vi "Generate_WayPoints_Hopping_LineScan.vi"(11 "Input Cluster":T2={"Scan Rate (um/s)"=15.0, "X Start"=15.0, "X End"=15.0, "Y Start"=15.0, "Y End"=15.0, " Z Start"=15.0, "HoppingDistance"=1.0, "V"=15.0, "Z End"=15.0, "Approach Rate Hopping (um/s)"=15.0, "Retract Rate (um/s)"=15.0, "V 2"=15.0, "Approach Rate (um/s)"=15.0}) -> (0 "output cluster":T1)   [LabVIEW 2023]
uses:
  TypeDefs/WayPointCluster.ctl
  User_Vi/Settings.vi
panel:
  out "Numeric":i32
  in  "WayPointCluster":T1
  out "Y  P":dbl
  out "X  P":dbl
  out "HoppingDistanceX":dbl
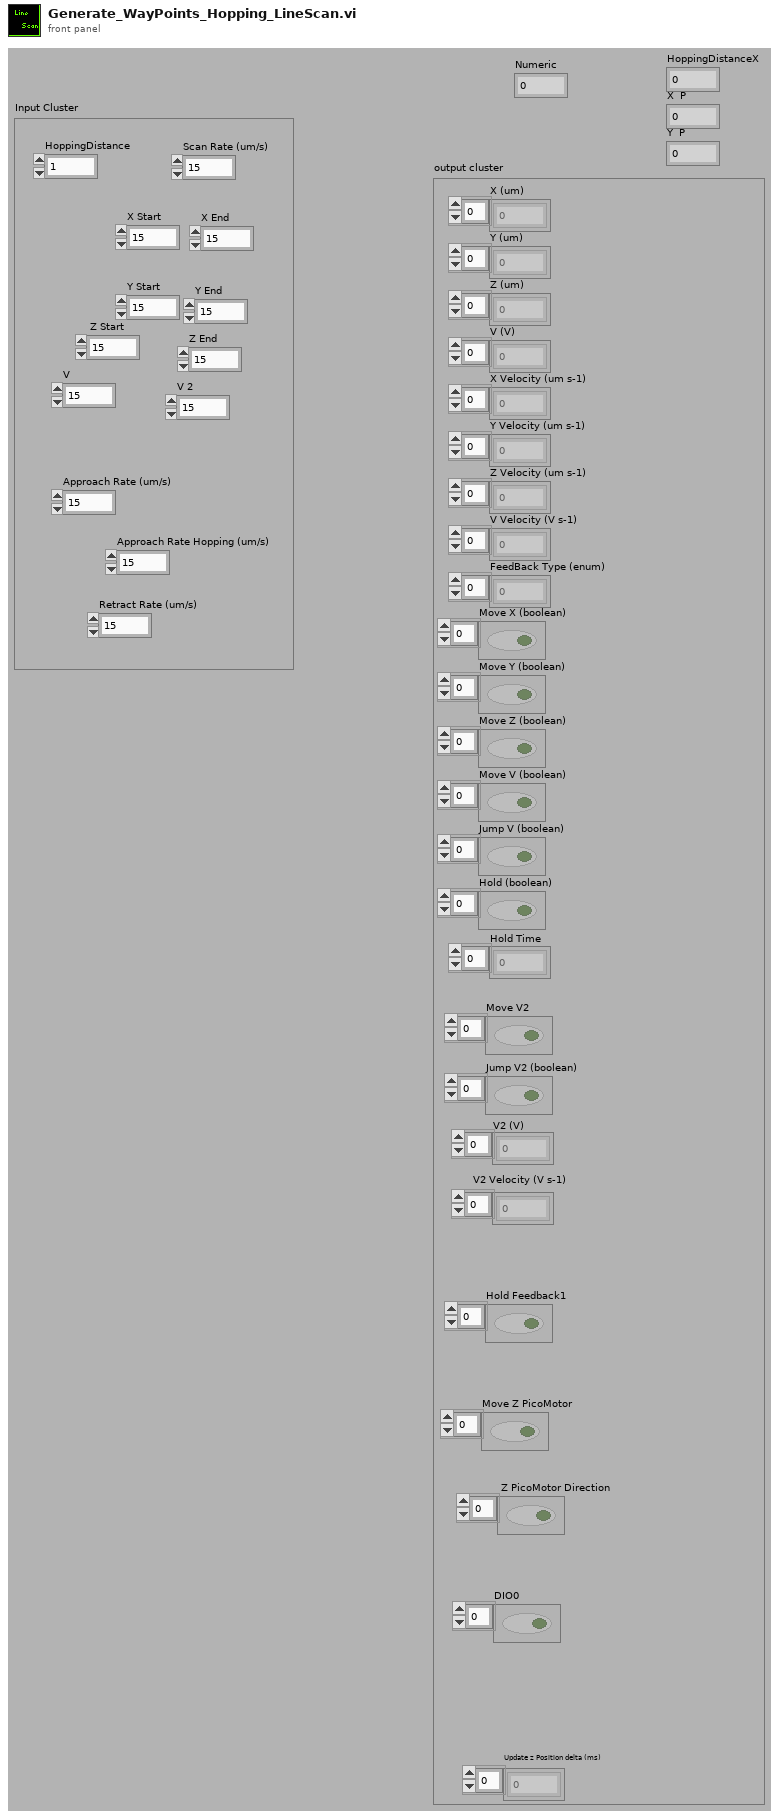
[diagram p1: front panel]
types:
  T1 = typedef "WayPointCluster.ctl" = cluster{"X (um)":dbl[], "Y (um)":dbl[], "Z (um)":dbl[], "V (V)":dbl[], "X Velocity (um s-1)":dbl[], "Y Velocity (um s-1)":dbl[], "Z Velocity (um s-1)":dbl[], "V Velocity (V s-1)":dbl[], "FeedBack Type (enum)":u16[], "Move X (boolean)":bool[], "Move Y (boolean)":bool[], "Move Z (boolean)":bool[], "Move V (boolean)":bool[], "Jump V (boolean)":bool[], "Hold (boolean)":bool[], "Hold Time":u32[], "V2 (V)":dbl[], "Move V2":bool[], "V2 Velocity (V s-1)":dbl[], "Jump V2 (boolean)":bool[], "Update z Position delta (ms)":i16[], "Hold Feedback1":bool[], "Move Z PicoMotor":bool[], " Z PicoMotor Direction":bool[], "DIO0":bool[]}
  T2 = cluster{"Scan Rate (um/s)":dbl, "X Start":dbl, "X End":dbl, "Y Start":dbl, "Y End":dbl, " Z Start":dbl, "HoppingDistance":dbl, "V":dbl, "Z End":dbl, "Approach Rate Hopping (um/s)":dbl, "Retract Rate (um/s)":dbl, "V 2":dbl, "Approach Rate (um/s)":dbl}
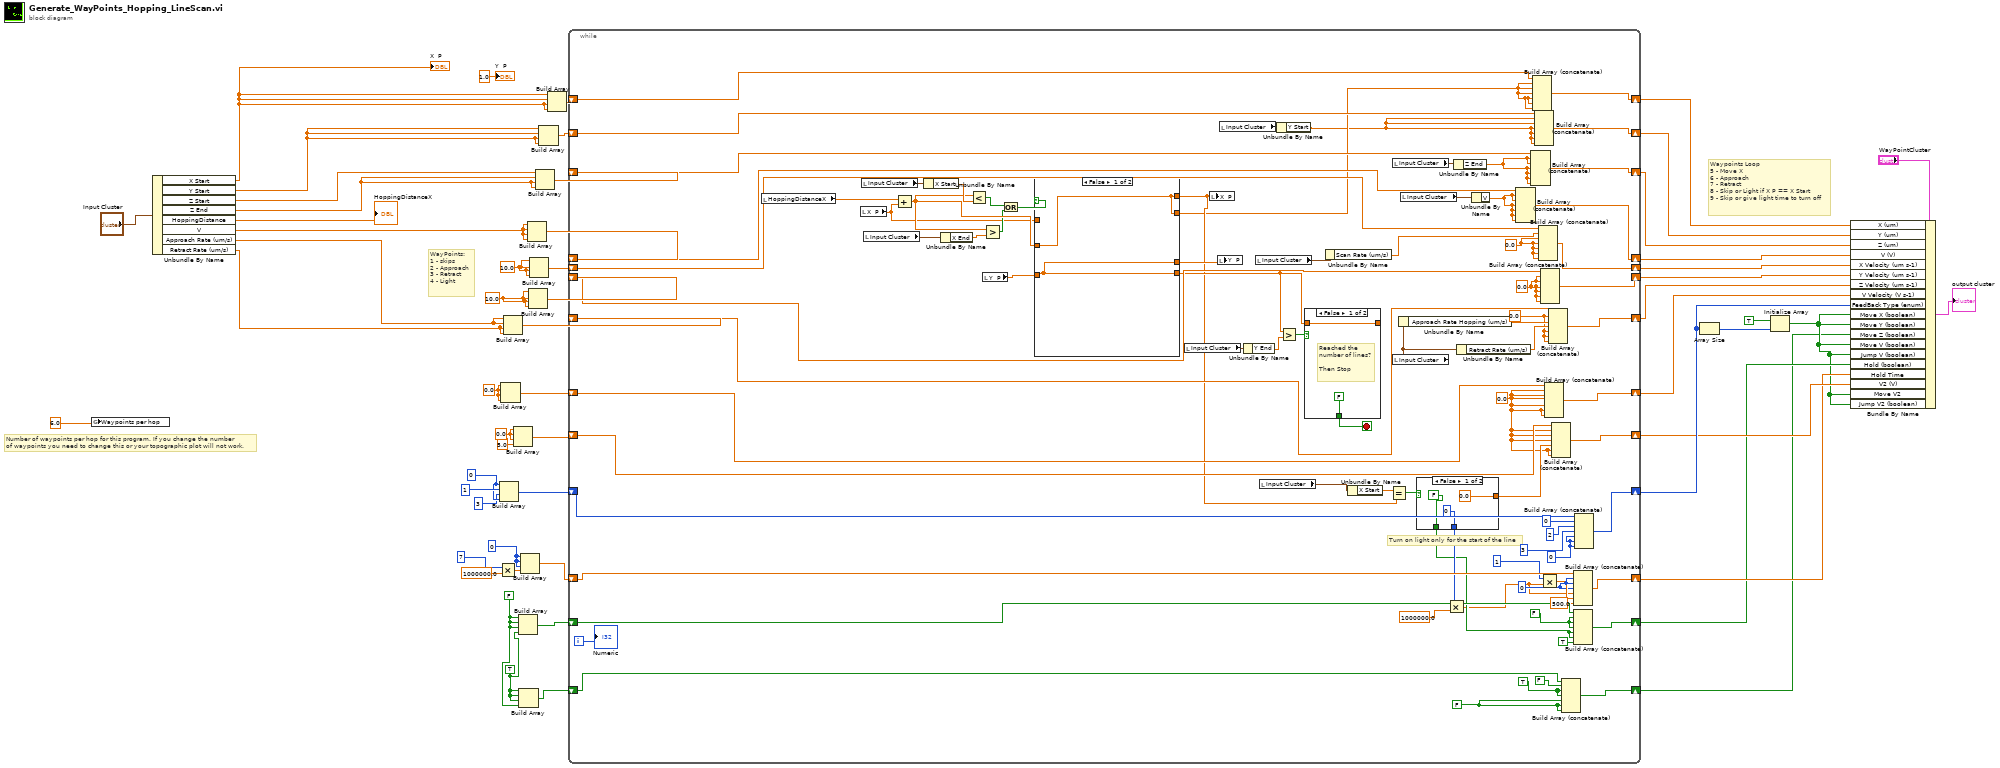
[diagram p0: block diagram]
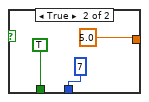
[diagram p2: hidden frame]
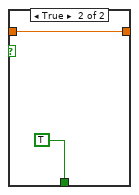
[diagram p3: hidden frame]
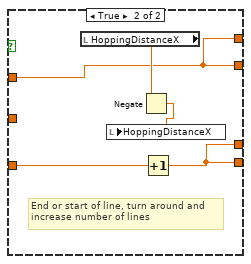
[diagram p4: hidden frame]
diagram:
  w19 = TRUE
  w20 = FALSE
  w28 = u16 0 ("element")
  w16 = 0.0 ("element")
  w17 = u16 0 ("element")
  w12 = 10.0 ("element")
  w13 = 10.0 ("element")
  w15 = 0.0 ("element")
  # "Number of waypoints per hop for this program. If you change the number\nof waypoints you need to change this or your topographic plot will not work."
  # "Waypoints Loop\n5 - Move X\n6 - Approach\n7 - Retract\n8 - Skip or Light if X P == X Start\n9 - Skip or give light time to turn off"
  # "WayPoints:\n1 - skips\n2 - Approach\n3 - Retract\n4 - Light"
  n1 = global write "Settings.vi" "Waypoints per hop"(6.0) -> ()
  n2 = Unbundle By Name("Input Cluster") -> ("X Start"=w8:dbl, "Y Start"=w7:dbl, "Z Start"=w37:dbl, "Z End"=w9:dbl, "HoppingDistance"=→"HoppingDistanceX":dbl, "V"=w11:dbl, "Approach Rate (um/s)"=w34:dbl, "Retract Rate (um/s)"=w14:dbl)
  "X  P" <- w8
  n3 = Multiply(x=u16 7 ("element"), y=1000000.0) -> (x*y=w18:dbl)
  n4 = Build Array(w17, u16 1 ("element"), u16 3 ("element"), w17) -> (w40:u16[])
  n5 = Build Array(w15, w15, w15, w15) -> (w30:dbl[])
  n6 = Build Array(w34, w34, w14, w14) -> (w43:dbl[])
  n7 = Build Array(w16, w16, w16, 5.0 ("element")) -> (w29:dbl[])
  n8 = Build Array(w20, w20, w20, w19) -> (w24:bool[])
  n9 = Build Array(w19, w19, w19, w20) -> (w22:bool[])
  n10 = Build Array(w28, w28, w28, w18) -> (w27:dbl[])
  n11 = Build Array(w11, w11, w11, w11) -> (w48:dbl[])
  n12 = Build Array(w13, w13, w13, w13) -> (w45:dbl[])
  n13 = Build Array(w12, w12, w12, w12) -> (w46:dbl[])
  n14 = Build Array(w37, w9, w9, w9) -> (w50:dbl[])
  n15 = Build Array(w7, w7, w7, w7) -> (w51:dbl[])
  n16 = Build Array(w8, w8, w8, w8) -> (w53:dbl[])
  n17 = while {
    shift-right: [w135] -> w52
    shift-left: w53 -> [w136]
    shift-right: [w127] -> w38
    shift-left: w51 -> [w118]
    shift-right: [w126] -> w49
    shift-left: w50 -> [w134]
    shift-right: [w125] -> w47
    shift-left: w48 -> [w133]
    shift-right: [w124] -> w4
    shift-left: w46 -> [w132]
    shift-right: [w100] -> w44
    shift-left: w45 -> [w131]
    shift-right: [w123] -> w42
    shift-left: w43 -> [w130]
    shift-right: [w122] -> w41
    shift-left: w30 -> [w129]
    shift-right: [w121] -> w36
    shift-left: w40 -> [w128]
    shift-right: [w95] -> w31
    shift-left: w29 -> [w90]
    shift-right: [w88] -> w26
    shift-left: w27 -> [w89]
    shift-right: [w87] -> w25
    shift-left: w24 -> [w85]
    shift-right: [w81] -> w21
    shift-left: w22 -> [w80]
    i -> [w83]
    stop <- w108 stop-if-true
    w60 = u16 0 ("element")
    w57 = FALSE
    w82 = TRUE
    w86 = FALSE
    w75 = u16 0 ("element")
    w63 = 0.0 ("element")
    w64 = 0.0 ("element")
    w61 = 0.0 ("element")
    w62 = 0.0 ("element")
    # "Turn on light only for the start of the line"
    n18 = local read "HoppingDistanceX"() -> (w101:dbl)
    n19 = local read "X  P"() -> (w102:dbl)
    n20 = local read "Input Cluster"() -> (w138:T2)
    n21 = local read "Input Cluster"() -> (w137:T2)
    n22 = Add(x=w101, y=w102) -> (x+y=w114:dbl)
    n23 = Unbundle By Name(w138) -> ("X Start"=w117:dbl)
    n24 = Unbundle By Name(w137) -> ("X End"=w115:dbl)
    n25 = Less?(x=w114, y=w117) -> (x < y?=w116:bool)
    n26 = local read "Y  P"() -> (w74:dbl)
    n27 = Greater?(x=w114, y=w115) -> (0:w113:bool)
    n28 = Or(x=w116, y=w113) -> (x .or. y?=w112:bool)
    n29 = case shown="False" w112 {
      tunnel: w114 -> [w150 _]
      tunnel: [w150 w153] -> w68
      tunnel: w102 -> [_ w153]
      tunnel: [w149 w152] -> w107
      tunnel: [w149 w152] -> w106
      tunnel: [w150 w153] -> w79
      tunnel: w74 -> [w149 w151]
      frame False {
      }
      frame True {
        # "End or start of line, turn around and \nincrease number of lines"
        n30 = local read "HoppingDistanceX"() -> (w155:dbl)
        n31 = Negate(x=w155) -> (-x=w154:dbl)
        n32 = local write "HoppingDistanceX"(w154) -> ()
        n33 = Increment(x=w151) -> (x+1=w152:dbl)
      }
    }
    n34 = local read "Input Cluster"() -> (w111:T2)
    n35 = local write "X  P"(w79) -> ()
    n36 = local write "Y  P"(w106) -> ()
    n37 = local read "Input Cluster"() -> (w96:T2)
    n38 = Unbundle By Name(w111) -> ("Y End"=w110:dbl)
    n39 = local read "Input Cluster"() -> (w70:T2)
    n40 = local read "Input Cluster"() -> (w93:T2)
    n41 = Unbundle By Name(w96) -> ("Y Start"=w67:dbl)
    n42 = Greater?(x=w107, y=w110) -> (0:w109:bool)
    n43 = case shown="False" w109 {
      tunnel: w107 -> [w146 w148]
      tunnel: [w146 w148] -> _
      tunnel: [FALSE TRUE] -> w108
      frame False {
        # "Reached the \nnumber of lines?\n\nThen Stop"
      }
      frame True {
      }
    }
    n44 = Unbundle By Name(w70) -> ("Scan Rate (um/s)"=w69:dbl)
    n45 = Unbundle By Name(w93) -> ("X Start"=w91:dbl)
    n46 = Equal?(x=w91, y=w79) -> (x = y?=w92:bool)
    n47 = local read "Input Cluster"() -> (w120:T2)
    n48 = local read "Input Cluster"() -> (w99:T2)
    n49 = Unbundle By Name(w99) -> ("Approach Rate Hopping (um/s)"=w103:dbl)
    n50 = local read "Input Cluster"() -> (w119:T2)
    n51 = case shown="False" w92 {
      tunnel: [0.0 ("element") 5.0 ("element")] -> w94
      tunnel: [FALSE TRUE] -> w78
      tunnel: [i64 0 ("element") i64 7 ("element")] -> w84
      frame False {
      }
      frame True {
      }
    }
    n52 = Multiply(x=w84, y=1000000.0) -> (x*y=w72:dbl)
    n53 = Unbundle By Name(w120) -> ("Z End"=w66:dbl)
    n54 = Unbundle By Name(w99) -> ("Retract Rate (um/s)"=w97:dbl)
    n55 = Unbundle By Name(w119) -> ("V"=w65:dbl)
    n56 = Build Array (concatenate)(w133, w65, w65, w65, w65, w65, w65) -> (w125:dbl[])
    n57 = Build Array (concatenate)(w134, w66, w66, w66, w66, w66, w66) -> (w126:dbl[])
    n58 = Build Array (concatenate)(w136, w68, w68, w68, w68, w68, w68) -> (w135:dbl[])
    n59 = Build Array (concatenate)(w118, w67, w67, w67, w67, w67, w67) -> (w127:dbl[])
    n60 = Build Array (concatenate)(w132, w69, w64, w64, w64, w64, w64) -> (w124:dbl[])
    n61 = Build Array (concatenate)(w131, w63, w63, w63, w63, w63, w63) -> (w100:dbl[])
    n62 = Multiply(x=i64 1 ("element"), y=w72) -> (x*y=w77:dbl)
    n63 = Build Array (concatenate)(w129, w61, w61, w61, w61, w61, w61) -> (w122:dbl[])
    n64 = Build Array (concatenate)(w130, w62, w103, w97, w62, w62, w62) -> (w123:dbl[])
    n65 = Build Array (concatenate)(w90, w61, w61, w61, w94, w61, w61) -> (w95:dbl[])
    n66 = Build Array (concatenate)(w80, FALSE, w82, w82, w57, w57, w57) -> (w81:bool[])
    n67 = Build Array (concatenate)(w89, w75, w75, w75, w72, w77, 500.0 ("element")) -> (w88:dbl[])
    n68 = Build Array (concatenate)(w85, w86, w86, w86, w78, w78, TRUE ("element")) -> (w87:bool[])
    n69 = Build Array (concatenate)(w128, u16 0 ("element"), u16 2 ("element"), u16 3 ("element"), w60, w60, w60) -> (w121:u16[])
    "Numeric" <- w83
  }
  n70 = Array Size(array=w36) -> (size(s)=w39:i32)
  n71 = Initialize Array(TRUE, w39) -> (w23:bool[])
  n72 = Bundle By Name(cluster="WayPointCluster", "X (um)"=w52, "Y (um)"=w38, "Z (um)"=w49, "V (V)"=w47, "X Velocity (um s-1)"=w4, "Y Velocity (um s-1)"=w44, "Z Velocity (um s-1)"=w42, "V Velocity (V s-1)"=w41, "FeedBack Type (enum)"=w36, "Move X (boolean)"=w23, "Move Y (boolean)"=w23, "Move Z (boolean)"=w21, "Move V (boolean)"=w23, "Jump V (boolean)"=w23, "Hold (boolean)"=w25, "Hold Time"=w26, "V2 (V)"=w31, "Move V2"=w23, "Jump V2 (boolean)"=w23) -> (→"output cluster":T1)
  "Y  P" <- 1.0 ("Y  P")
